vi "Arm_Move.vi"(8 "Enum":enum16{"1", "2", "3", "4", ""}(ring), 9 "Theta 3 Actual":dbl, 10 "Theta 2 Actual":dbl, 11 "Theta 1 Actual":dbl) -> (0 "Too Far Out":bool, 1 "Theta 3 Set":dbl, 2 "Theta 2 Set":dbl, 3 "Theta 1 Set":dbl)   [LabVIEW 2017]
panel:
  out "X Out":dbl
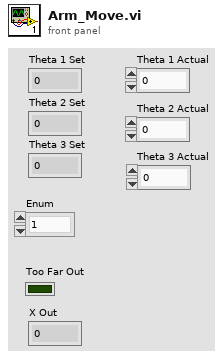
[diagram p1: front panel]
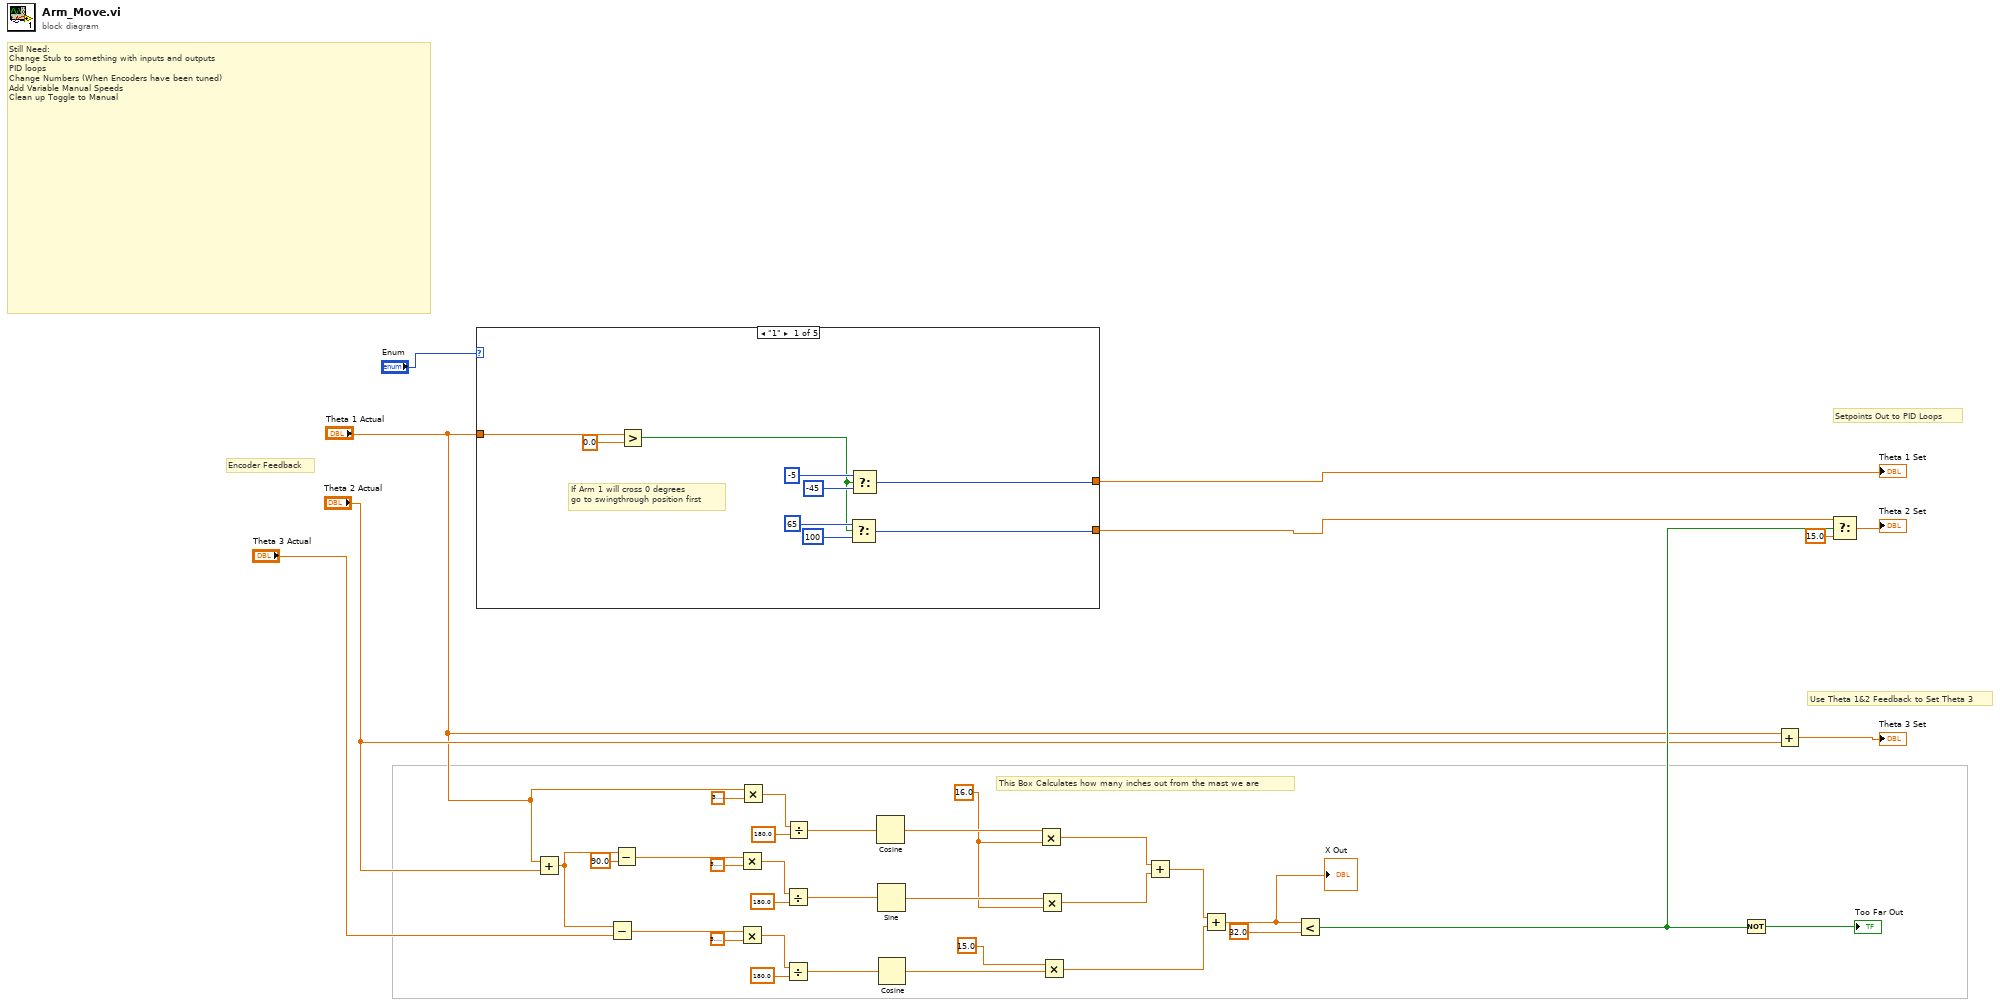
[diagram p0: block diagram]
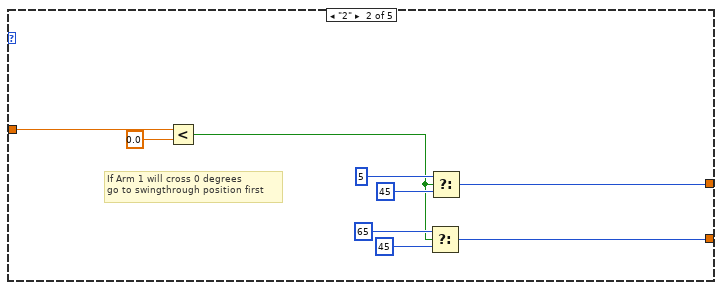
[diagram p2: hidden frame]
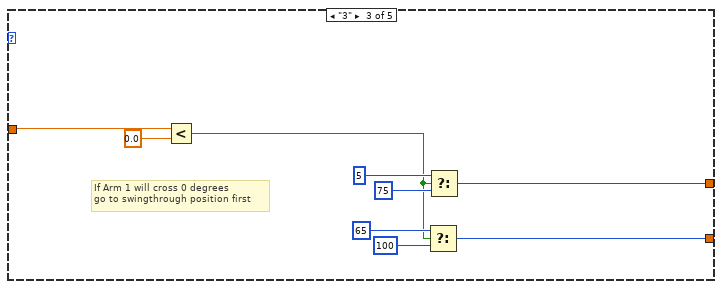
[diagram p3: hidden frame]
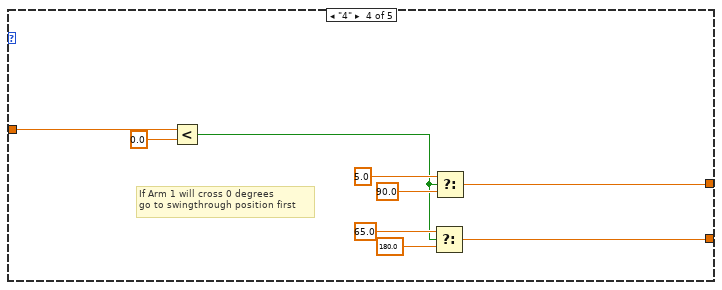
[diagram p4: hidden frame]
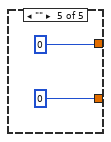
[diagram p5: hidden frame]
diagram:
  w4 = 16.0
  # "This Box Calculates how many inches out from the mast we are"
  # "Use Theta 1&2 Feedback to Set Theta 3"
  # "Still Need:\nChange Stub to something with inputs and outputs\nPID loops\nChange Numbers (When Encoders have been tuned) \nAdd Variable Manual Speeds\nClean up Toggle to Manual"
  # "Encoder Feedback"
  # "Setpoints Out to PID Loops"
  n1 = case shown="\"1\"" "Enum" {
    tunnel: [w39 w49 w58 w67 0] -> w3
    tunnel: [w40 w48 w57 w66 0] -> w2
    tunnel: "Theta 1 Actual" -> [w46 w50 w59 w68 _]
    frame "1" {
      # "If Arm 1 will cross 0 degrees\ngo to swingthrough position first"
      n2 = Greater?(x=w46, y=0.0) -> (0:w41:bool)
      n3 = Select(t=65, s=w41, f=100) -> (s? t:f=w40:i32)
      n4 = Select(t=-5, s=w41, f=-45) -> (s? t:f=w39:i32)
    }
    frame "2" {
      # "If Arm 1 will cross 0 degrees\ngo to swingthrough position first"
      n5 = Less?(x=w50, y=0.0) -> (x < y?=w51:bool)
      n6 = Select(t=65, s=w51, f=45) -> (s? t:f=w48:i32)
      n7 = Select(t=5, s=w51, f=45) -> (s? t:f=w49:i32)
    }
    frame "3" {
      # "If Arm 1 will cross 0 degrees\ngo to swingthrough position first"
      n8 = Less?(x=w59, y=0.0) -> (x < y?=w60:bool)
      n9 = Select(t=65, s=w60, f=100) -> (s? t:f=w57:i32)
      n10 = Select(t=5, s=w60, f=75) -> (s? t:f=w58:i32)
    }
    frame "4" {
      # "If Arm 1 will cross 0 degrees\ngo to swingthrough position first"
      n11 = Less?(x=w68, y=0.0) -> (x < y?=w69:bool)
      n12 = Select(t=65.0, s=w69, f=180.0) -> (s? t:f=w66:dbl)
      n13 = Select(t=5.0, s=w69, f=90.0) -> (s? t:f=w67:dbl)
    }
    frame "" {
    }
  }
  "Theta 1 Set" <- w3
  n14 = Add(x="Theta 1 Actual", y="Theta 2 Actual") -> (x+y=w34:dbl)
  n15 = Subtract(x=w34, y="Theta 3 Actual") -> (x-y=w15:dbl)
  n16 = Subtract(x=w34, y=90.0) -> (x-y=w16:dbl)
  n17 = Multiply(x=w16, y=3.141592653589793) -> (x*y=w22:dbl)
  n18 = Multiply(x=w15, y=3.141592653589793) -> (x*y=w19:dbl)
  n19 = Multiply(x="Theta 1 Actual", y=3.141592653589793) -> (x*y=w25:dbl)
  n20 = Divide(x=w22, y=180.0) -> (x/y=w17:dbl)
  n21 = Divide(x=w19, y=180.0) -> (x/y=w14:dbl)
  n22 = Divide(x=w25, y=180.0) -> (x/y=w18:dbl)
  n23 = Cosine(x=w18) -> (cos(x)=w37:dbl)
  n24 = Sine(x=w17) -> (sin(x)=w36:dbl)
  n25 = Cosine(x=w14) -> (cos(x)=w32:dbl)
  n26 = Multiply(x=w37, y=w4) -> (x*y=w31:dbl)
  n27 = Multiply(x=w36, y=w4) -> (x*y=w30:dbl)
  n28 = Multiply(x=15.0, y=w32) -> (x*y=w29:dbl)
  n29 = Add(x=w31, y=w30) -> (x+y=w28:dbl)
  n30 = Add(x=w28, y=w29) -> (x+y=w12:dbl)
  "X Out" <- w12
  n31 = Less?(x=w12, y=32.0 ("x")) -> (x < y?=w11:bool)
  n32 = Not(x=w11) -> (.not. x?=→"Too Far Out":bool)
  n33 = Add(x="Theta 1 Actual", y="Theta 2 Actual") -> (x+y=→"Theta 3 Set":dbl)
  n34 = Select(t=w2, s=w11, f=15.0) -> (s? t:f=→"Theta 2 Set":dbl)
